vi "Configuration - DMM Properties FGV.vi"(8 "error in (no error)":errorcluster, 11 "Configuration Group of Channels Ref In":T1 format="%.0x") -> (0 "error out":errorcluster, 3 "Configuration Group of Channels Ref Out":T1 format="%.0x")   [LabVIEW 2015, in "DMM-SWITCH-ScanList System Explorer.lvlib"]
uses:
  DMM-SWITCH-ScanList System Explorer.lvlib
  <vilib>/NI Veristand/Custom Device API/Custom Device Item Ref.ctl
  <vilib>/NI Veristand/Custom Device API/Custom Device Channel.ctl
  <vilib>/NI Veristand/Custom Device API/Custom Device Channel Type.ctl
  Shared/Constants.vi
  <vilib>/NI Veristand/Custom Device API/Set Item Property (String).vi
  <vilib>/NI Veristand/Custom Device API/Set Item Property (U16).vi
  <vilib>/NI Veristand/Custom Device API/Set Item Property (Double).vi
  <vilib>/NI Veristand/Custom Device API/Custom Device API.lvlib
  Shared/DMM-SWITCH-ScanList Shared.lvlib
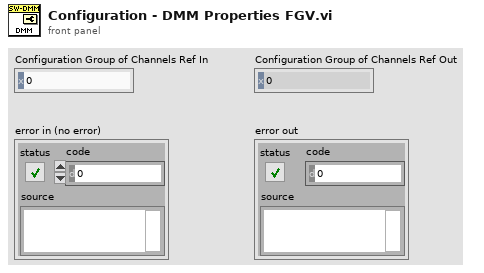
[diagram p1: front panel]
types:
  T1 = typedef "Custom Device API.lvlib/Custom Device Item Ref.ctl" = u64
  T2 = typedef "Custom Device API.lvlib/Custom Device Channel.ctl" = cluster{"Type":T3, "Units":string, "Default Value":dbl, "Faultable":bool, "Scalable":bool}
  T3 = typedef "Custom Device API.lvlib/Custom Device Channel Type.ctl" = enum16{"Input", "Output"}
  T4 = typedef "niDMM Function.ctl" = enum16{"DC Volts", "AC Volts", "DC Current", "AC Current", "2-wire Resistance", "4-wire Resistance", "Diode", "Frequency", "Period", "AC Volts DC Coupled", "Capacitance", "Inductance", "Temperature"}
  T5 = typedef "niDMM Resolution in Digits.ctl" = dbl
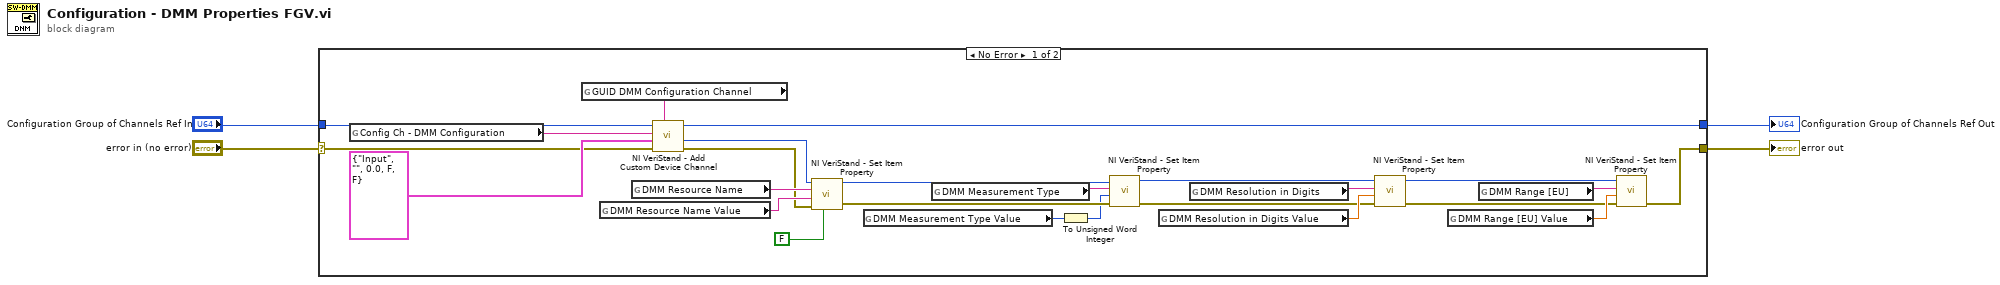
[diagram p0: block diagram]
diagram:
  n1 = case shown="No Error" "error in (no error)" {
    selector: "error in (no error)" -> [w6 w30]
    tunnel: [w17 w30] -> w4
    tunnel: [w8 w31] -> w3
    tunnel: "Configuration Group of Channels Ref In" -> [w7 w31]
    frame No Error {
      n2 = global read "Constants.vi" "Config Ch - DMM Configuration"() -> (w5:string)
      n3 = global read "Constants.vi" "GUID DMM Configuration Channel"() -> (w25:string)
      n4 = global read "Constants.vi" "DMM Resource Name Value"() -> (w21:string)
      n5 = global read "Constants.vi" "DMM Resource Name"() -> (w26:string)
      n6 = call <vilib>:"NI VeriStand - Add Custom Device Channel.vi"("GUID (Default Channel)"=w25, "error in (no error)"=w6, "Channel"=T2 {"Type"=enum."Input", "Units"="", "Default Value"=0.0, "Faultable"=FALSE, "Scalable"=FALSE}, "Channel Name"=w5, "Parent Ref in"=w7) -> ("error out"=w18:errorcluster, "Channel Ref"=w9:T1, "Parent Ref out"=w8:T1)  [unwired: 3 in, 1 out]
      n7 = call-poly <vilib>:"NI VeriStand - Set Item Property.vi"("Binary String (T)"=FALSE, "error in (no error)"=w18, "Value"=w21, "Property Name"=w26, "Item Ref in"=w9) -> ("error out"=w11:errorcluster, "Item Ref out"=w12:T1)  [unwired: 4 in, 1 out]
      n8 = global read "Constants.vi" "DMM Measurement Type Value"() -> (w22:T4)
      n9 = global read "Constants.vi" "DMM Measurement Type"() -> (w27:string)
      n10 = To Unsigned Word Integer(number=w22) -> (unsigned 16bit integer=w10:u16)
      n11 = call-poly <vilib>:"NI VeriStand - Set Item Property.vi"("error in (no error)"=w11, "Value"=w10, "Property Name"=w27, "Item Ref in"=w12) -> ("error out"=w14:errorcluster, "Item Ref out"=w13:T1)  [unwired: 5 in, 1 out]
      n12 = global read "Constants.vi" "DMM Resolution in Digits Value"() -> (w23:T5)
      n13 = global read "Constants.vi" "DMM Resolution in Digits"() -> (w28:string)
      n14 = call-poly <vilib>:"NI VeriStand - Set Item Property.vi"("error in (no error)"=w14, "Value"=w23, "Property Name"=w28, "Item Ref in"=w13) -> ("error out"=w16:errorcluster, "Item Ref out"=w15:T1)  [unwired: 5 in, 1 out]
      n15 = global read "Constants.vi" "DMM Range [EU] Value"() -> (w24:dbl)
      n16 = global read "Constants.vi" "DMM Range [EU]"() -> (w29:string)
      n17 = call-poly <vilib>:"NI VeriStand - Set Item Property.vi"("error in (no error)"=w16, "Value"=w24, "Property Name"=w29, "Item Ref in"=w15) -> ("error out"=w17:errorcluster)  [unwired: 5 in, 2 out]
    }
    frame Error {
    }
  }
  "error out" <- w4
  "Configuration Group of Channels Ref Out" <- w3
